vi "Actor Core.vi"(8 "error in":errorcluster, 11 "Nested in":refnum<class "Test Application Controller.lvclass">) -> (0 "error out":errorcluster, 3 "Actor out":refnum<class "Actor.lvclass">)   [LabVIEW 2017, in "Test Application Controller.lvlib" / "Test Application Controller.lvclass"]
doc: "(<B>Filename</B>: Actor Framework.lvlib:Actor.lvclass:Actor Core.vi)\n\nReceives messages to the actor, reacts to them, and initiates any error handling that may shut the actor down.\n\nDescendant classes may override this VI to append parallel tasks for the actor to complete while it handles messages. Overrides use the Call Parent Method node."
uses:
  Test Application Controller.lvclass
  C:/Program Files (x86)/National Instruments/LabVIEW 2017/vi.lib/ActorFramework/Actor/Actor.lvclass
  <vilib>/ActorFramework/Actor/Actor.lvclass
  <vilib>/ActorFramework/Actor/Actor.lvclass/Actor.ctl
  <vilib>/ActorFramework/Message Enqueuer/Message Enqueuer.lvclass/Message Enqueuer.ctl
  Test Application Controller.lvclass/Test Application Controller.ctl
  Test Application Controller Messages/Update UI Status String Msg/Update UI Status String Msg.lvclass/Update UI Status String Msg.ctl
  Test Application Controller Messages/Launch Test Msg/Launch Test Msg.lvclass/Launch Test Msg.ctl
  <vilib>/ActorFramework/Message Enqueuer/Init from Existing Queue.vi
  <vilib>/ActorFramework/Message Enqueuer/Enqueue.vi
  <vilib>/ActorFramework/Stop Msg/Stop Msg.lvclass
  C:/Program Files (x86)/National Instruments/LabVIEW 2017/vi.lib/ActorFramework/Message/Message.lvclass
  Test Application Controller Messages/Update UI Status String Msg/Update UI Status String Msg.lvclass
  Test Application Controller Messages/Launch Test Msg/Launch Test Msg.lvclass
  <vilib>/ActorFramework/Message Priority Queue/Priority Enqueue.vi
  <vilib>/ActorFramework/Message Enqueuer/Message Enqueuer.lvclass
panel:
  out "Generate Report":bool
  out "Stop Test":bool
  out "Tests to Execute":string[](array[string])
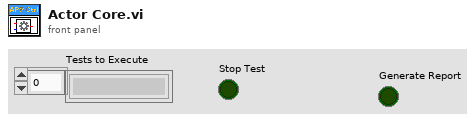
[diagram p1: front panel]
types:
  T1 = cluster{"Stop":refnum<user-event>, "Tests to Execute":refnum<user-event>, "Stop Test":refnum<user-event>, "Generate Report":refnum<user-event>, "Status String":refnum<user-event>}
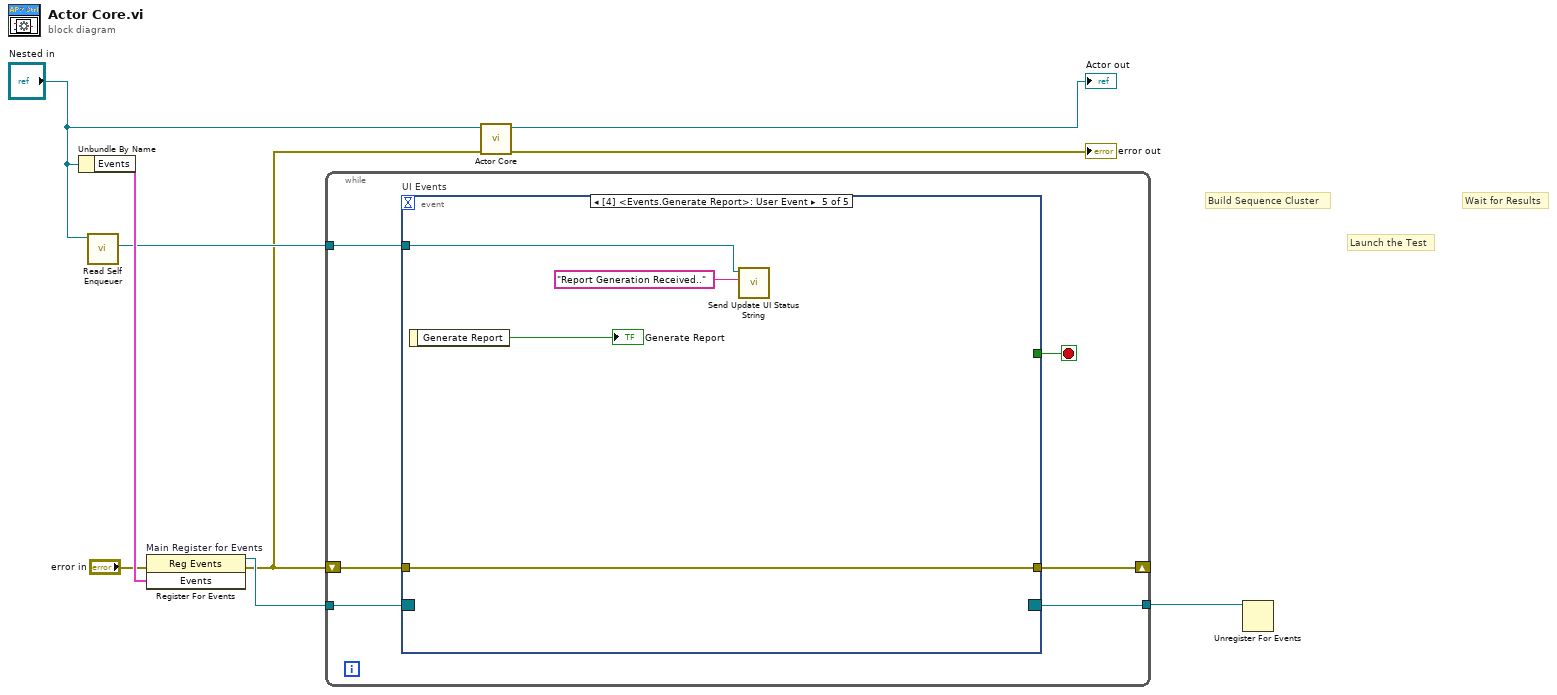
[diagram p0: block diagram]
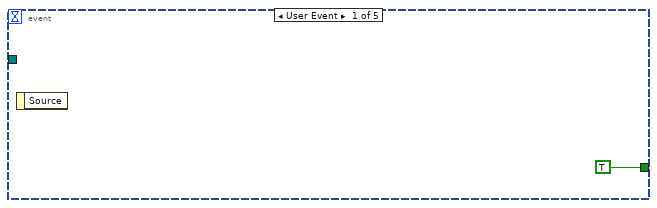
[diagram p2: hidden frame]
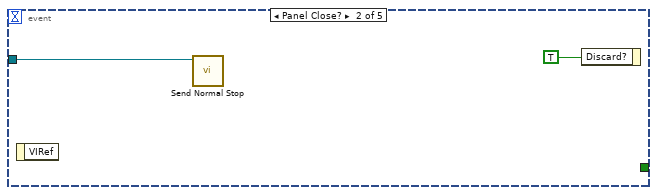
[diagram p3: hidden frame]
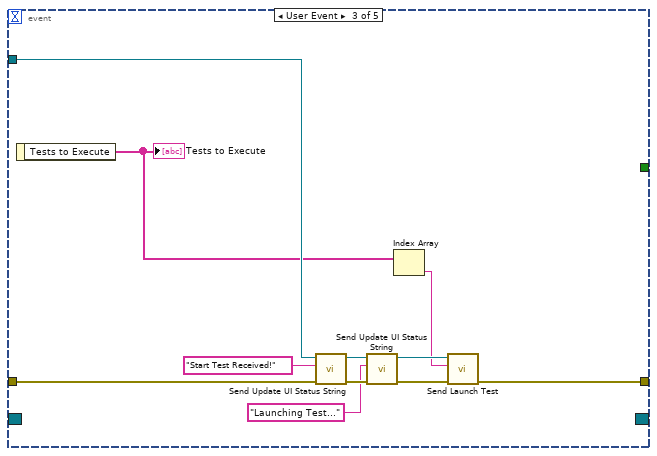
[diagram p4: hidden frame]
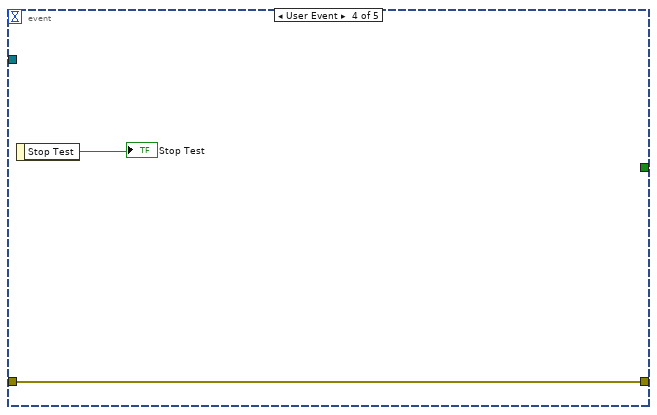
[diagram p5: hidden frame]
diagram:
  # "Wait for Results"
  # "Launch the Test"
  # "Build Sequence Cluster"
  n1 = Unbundle By Name("Nested in") -> ("Events"=w6:T1)
  n2 = call <vilib>:"Read Self Enqueuer.vi"("Actor"="Nested in") -> ("Self Enqueuer"=w4:refnum<class "Message Enqueuer.lvclass">)  [unwired: 10 in]
  n3 = register-events "Main Register for Events"(error in="error in", w6) -> (reference out=w7:refnum<event-registration>, error out=w1:errorcluster)  [unwired: 1 in]
  n4 = while {
    tunnel: w7 -> [w15]
    tunnel: [w13] -> w5
    tunnel: w4 -> [w12]
    shift-right: [w10] -> _
    shift-left: w1 -> [w11]
    stop <- w14 stop-if-true
    n5 = event "UI Events" shown="[4] <Events.Generate Report>: User Event" {
      selector: w15 -> [_ _ _ _ _]
      dyn-events: [_ _ _ _ _] -> w13
      timeout: _ -> [_ _ _ _ _]
      tunnel: [TRUE _ _ _ _] -> w14
      tunnel: w12 -> [_ w17 w29 _ w34]
      tunnel: w11 -> [_ _ w22 w30 w32]
      tunnel: [_ _ w21 w30 w32] -> w10
      event User Event {
        n6 = event-data() -> ()  [unwired: 1 in, 1 out]
      }
      event Panel Close? {
        n7 = event-data() -> ()  [unwired: 1 in, 1 out]
        n8 = call <vilib>:"Send Normal Stop.vi"("Message Enqueuer"=w17) -> ()  [unwired: 10 in, 1 out]
        n9 = event-data("Discard?"=TRUE) -> ()  [unwired: 1 in, 1 out]
      }
      event User Event {
        n10 = event-data() -> ("Tests to Execute"=w20:string[])  [unwired: 1 in]
        "Tests to Execute" <- w20
        n11 = call "Send Update UI Status String.vi"("error in (no error)"=w22, "Status"="Start Test Received!" ("message"), "Message Enqueuer"=w29) -> ("error out"=w27:errorcluster, "Message Enqueuer out"=w26:refnum<class "Message Enqueuer.lvclass">)  [unwired: 7 in]
        n12 = call "Send Update UI Status String.vi"("error in (no error)"=w27, "Status"="Launching Test..." ("message"), "Message Enqueuer"=w26) -> ("error out"=w23:errorcluster, "Message Enqueuer out"=w24:refnum<class "Message Enqueuer.lvclass">)  [unwired: 7 in]
        n13 = Index Array(array=w20) -> (element=w19:string)  [unwired: 1 in]
        n14 = call "Send Launch Test.vi"("error in (no error)"=w23, "Test Name"=w19, "Message Enqueuer"=w24) -> ("error out"=w21:errorcluster)  [unwired: 7 in, 1 out]
      }
      event User Event {
        n15 = event-data() -> ("Stop Test"=→"Stop Test":bool)  [unwired: 1 in]
      }
      event User Event {
        n16 = event-data() -> ("Generate Report"=→"Generate Report":bool)  [unwired: 1 in]
        n17 = call "Send Update UI Status String.vi"("Status"="Report Generation Received..", "Message Enqueuer"=w34) -> ()  [unwired: 8 in, 2 out]
      }
    }
  }
  n18 = call-parent "Actor Core.vi"("error in"=w1, "Actor in"="Nested in") -> ("error out"=→"error out":errorcluster, "Actor out"=→"Actor out":refnum<class "Actor.lvclass">)  [unwired: 8 in]
  n19 = Unregister For Events(event registration refnum=w5) -> ()  [unwired: 1 in, 1 out]
